vi "Get Type.vi"(11 "IntegerPanel in":refnum<class "IntegerPanel.lvclass">) -> (2 "Type":refnum<class "Type.lvclass">)   [LabVIEW 2020, in "Conditum-Tools.lvlib" / "IntegerPanel.lvclass"]
uses:
  IntegerPanel.lvclass
  Conditum-Clone/Columns/Type/Type.lvclass
  IntegerPanel.lvclass/IntegerPanel.ctl
  Conditum-Clone/Columns/Integer/Integer.lvclass
  C:/dev/lv20CE/lv-conditum-tools/Conditum-Clone/Columns/Type/Type.lvclass
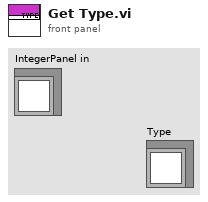
[diagram p1: front panel]
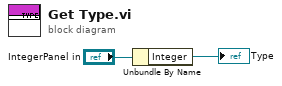
[diagram p0: block diagram]
diagram:
  n1 = Unbundle By Name("IntegerPanel in") -> ("Integer"=→"Type":refnum<class "Integer.lvclass">)
